vi "IV_sequential.vi"() -> ()   [LabVIEW 2013]
uses:
  InstrControl/Switching/Switching.lvclass
  QCtests/general_VIs/globals/QC_RunInformation.vi
  InstrControl/InstrControl.lvclass
panel:
  in  "Quit":bool
  in  "Continue":bool
  out "DB Serial Nos.":string[](array[string])
  in  "New Button":bool
  in  "Add Button":bool
  in  "Hardware Configurations":bool
  out "Channel Nos.":string[](array[string])
  # "Sensor QC: sequential IV"
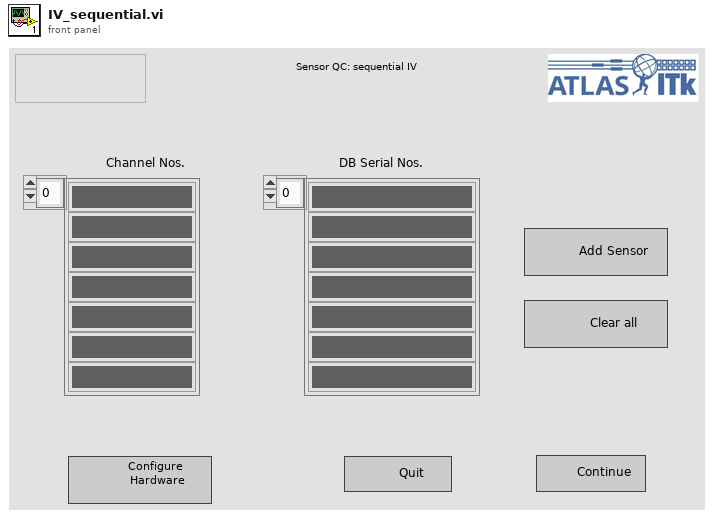
[diagram p1: front panel]
types:
  T1 = enum16{"Supply", "LCR", "Multimeter", "Switching"}
  T2 = cluster{"Institute":string, "Manufacturers":string[], "Devices":string[], "Serialnumbers Lookup DB":string, "Data directory":string, "Backup & screenshot directory":string, "List of known users":string[], "Measurement switch not used":bool, "Measurement Switch":string, "DUT Switch":string, "Rseries IV [MOhm]":string, "Rshunt IV [MOhm]":string, "Rseries CV [MOhm]":string, "DC blocking Cap [µF]":string, "Rseries LCR [MOhm]":string, "Rseries stability [MOhm]":string, "Rshunt stability [MOhm]":string, "Rseries striptest bias [MOhm]":string, "Rseries strip pinhole [MOhm]":string}
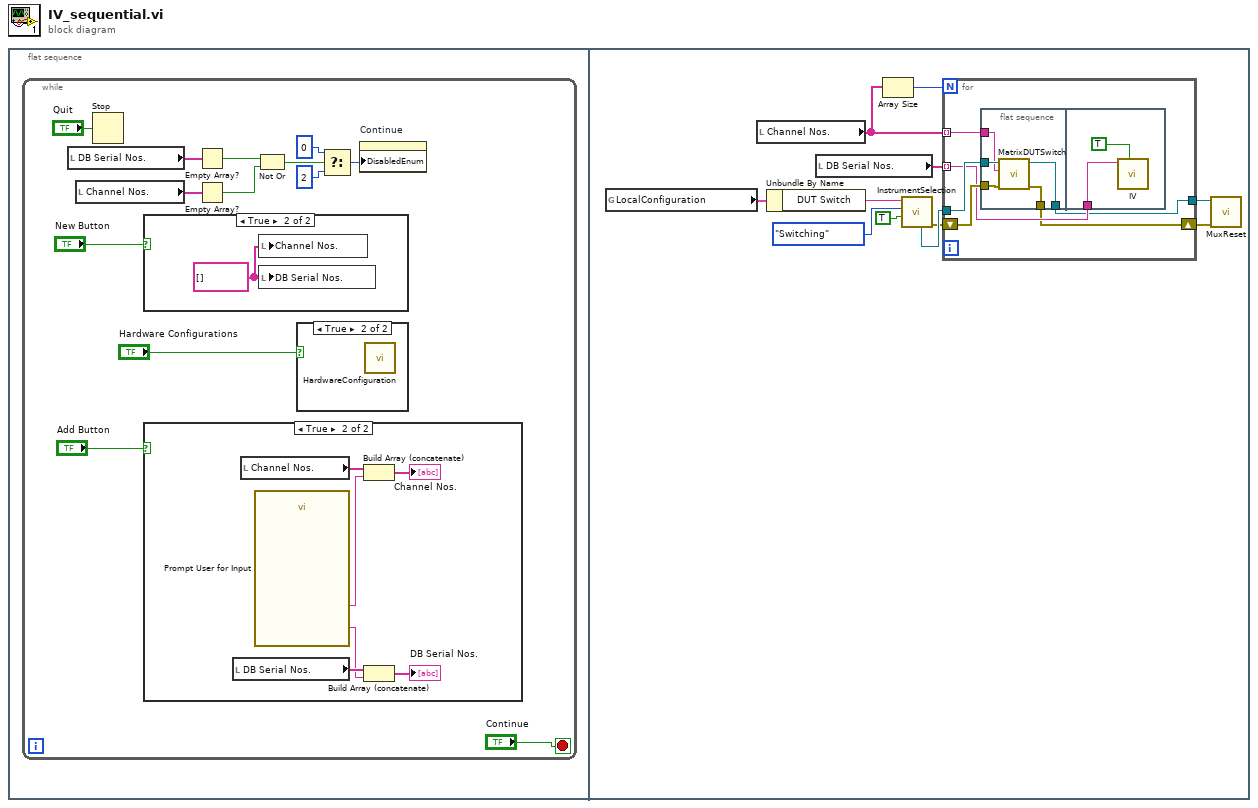
[diagram p0: block diagram]
diagram:
  n1 = flat-sequence {
    frame #0 {
      n2 = while {
        stop <- "Continue" stop-if-true
        n3 = local read "DB Serial Nos."() -> (w9:string[])
        n4 = local read "Channel Nos."() -> (w10:string[])
        n5 = Stop(stop? (T)="Quit") -> ()
        n6 = case shown="True" "New Button" {
          frame False {
          }
          frame True {
            w14 = string[] [] ("Channel Nos.")
            n7 = local write "Channel Nos."(w14) -> ()
            n8 = local write "DB Serial Nos."(w14) -> ()
          }
        }
        n9 = case shown="True" "Add Button" {
          frame False {
          }
          frame True {
            n10 = local read "DB Serial Nos."() -> (w17:string[])
            n11 = local read "Channel Nos."() -> (w20:string[])
            n12 = call "Prompt User for Input"() -> ("DB serial no."=w16:string, "channel no."=w18:string)  [unwired: 16 in, 2 out]
            n13 = Build Array (concatenate)(w20, w18) -> (→"Channel Nos.":string[])
            n14 = Build Array (concatenate)(w17, w16) -> (→"DB Serial Nos.":string[])
          }
        }
        n15 = Empty Array?(array=w9) -> (empty?=w8:bool)
        n16 = Empty Array?(array=w10) -> (empty?=w7:bool)
        n17 = Not Or(1:w7, 2:w8) -> (0:w3:bool)
        n18 = case shown="True" "Hardware Configurations" {
          frame False {
          }
          frame True {
            n19 = call "HardwareConfiguration.vi"() -> ()  [unwired: 11 in, 1 out]
          }
        }
        n20 = Select(t=0, s=w3, f=2) -> (s? t:f=w2:i32)
        n21 = property on="Continue" class="Bool"("DisabledEnum"=w2) -> ()  [unwired: 2 in, 2 out]
      }
    }
    frame #1 {
      n22 = global read "QC_RunInformation.vi" "LocalConfiguration"() -> (w31:T2)
      n23 = local read "Channel Nos."() -> (w25:string[])
      n24 = Unbundle By Name(w31) -> ("DUT Switch"=w30:string)
      n25 = local read "DB Serial Nos."() -> (w26:string[])
      n26 = Array Size(array=w25) -> (size(s)=w27:i32)
      n27 = call "InstrumentSelection.vi"("Verify GPIB address"=TRUE, "Instrument type"=T1."Switching", "Instrument name IN"=w30) -> ("error out"=w23:errorcluster, "Switching"=w24:refnum<class "Switching.lvclass">)  [unwired: 3 in, 4 out]
      n28 = for {
        N: w27 -> [_]
        tunnel: w26 -> [w34] mode=indexing
        tunnel: w25 -> [w36] mode=indexing
        tunnel: w24 -> [w37]
        tunnel: [w33] -> w22
        shift-right: [w32] -> w21
        shift-left: w23 -> [w35]
        n29 = flat-sequence {
          tunnel: w37 -> [w42]
          tunnel: w36 -> [w41]
          tunnel: w35 -> [w40]
          tunnel: [w39] -> w33
          tunnel: [w38] -> w32
          tunnel: w34 -> [w44]
          frame #0 {
            n30 = call-dynamic "MatrixDUTSwitch.vi"("error in (no error)"=w40, "Channel #"=w41, "Switching in"=w42) -> ("error out"=w38:errorcluster, "Switching out"=w39:refnum<class "Switching.lvclass">)  [unwired: 7 in]
          }
          frame #1 {
            n31 = call "IV.vi"("Run uninterrupted?"=TRUE, "DB Serial No. IN:"=w44) -> ()  [unwired: 4 in, 1 out]
          }
        }
      }
      n32 = call-dynamic "MuxReset.vi"("error in (no error)"=w21, "Switching in"=w22) -> ()  [unwired: 8 in, 2 out]
    }
  }
